vi "get desired keys.vi"(8 "error in":errorcluster, 11 "RTResourceUtilitzation configuration in":refnum<class "RTResourceUtilitzation configuration.lvclass">) -> (0 "error out":errorcluster, 2 "desired keys":string[](array[string]), 3 "RTResourceUtilitzation configuration out":refnum<class "RTResourceUtilitzation configuration.lvclass">)   [LabVIEW 2014, in "RTResourceUtilitzation configuration.lvclass"]
uses:
  RTResourceUtilitzation configuration.lvclass
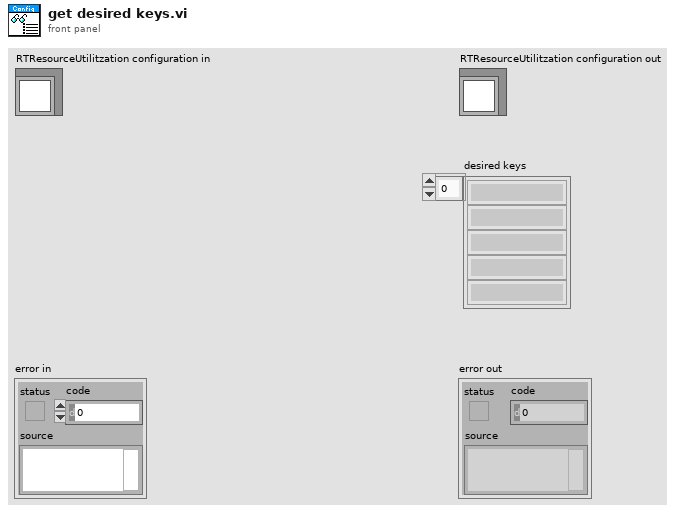
[diagram p1: front panel]
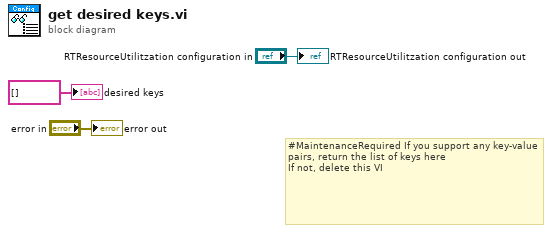
[diagram p0: block diagram]
diagram:
  # "#MaintenanceRequired If you support any key-value pairs, return the list of keys here\nIf not, delete this VI"
  "error out" <- "error in"
  "RTResourceUtilitzation configuration out" <- "RTResourceUtilitzation configuration in"
  "desired keys" <- string[] [] ("desired keys")
